vi "Subvi AO trigger.vi"(6 "EnableAsyncTrig":bool, 8 "FrameDelay_tick":u32, 9 "FirstFrameDelay_tick":u32, 10 "Reset":bool, 11 "Trigger":bool) -> (1 "IteratorDirection":bool, 3 "Stop":bool, 4 "Framecount":u16)   [LabVIEW 2017]
uses:
  GV AsyncTrigger.vi
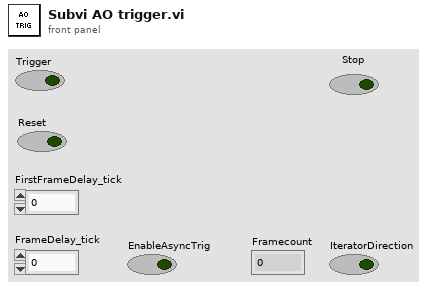
[diagram p1: front panel]
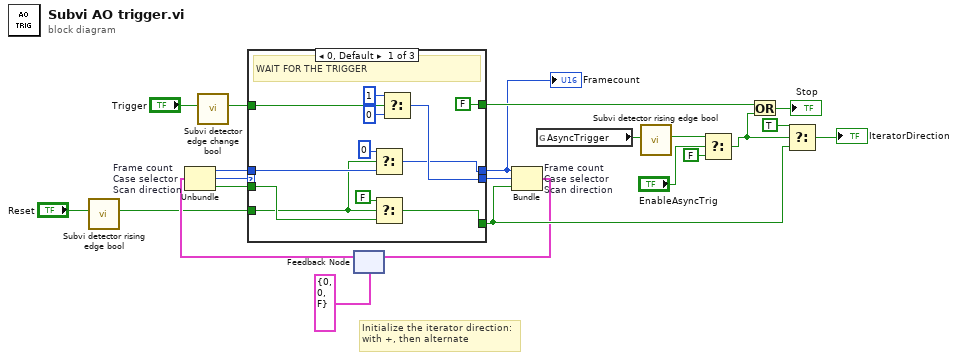
[diagram p0: block diagram]
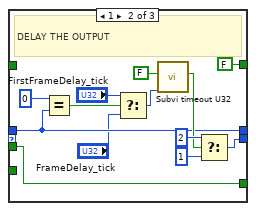
[diagram p2: hidden frame]
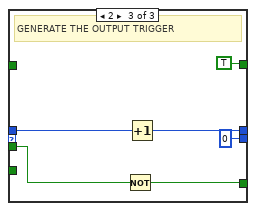
[diagram p3: hidden frame]
diagram:
  # "Initialize the iterator direction:\nwith +, then alternate"
  n1 = call "Subvi detector rising edge bool.vi"("Input"="Reset") -> ("Output"=w6:bool)  [unwired: 10 in]
  n2 = call "Subvi detector edge change bool.vi"("Input"="Trigger") -> ("Output"=w14:bool)  [unwired: 8 in]
  n3 = feedback #1(cluster{i16, "f":u8, bool} {0, "f"=0, FALSE}) -> (w12:cluster{u16, "f":u8, "t":bool})
  n4 = Unbundle "Frame count\nCase selector\nScan direction"(w12) -> (w11:u16, "f"=w9:u8, "t"=w10:bool)
  n5 = case shown="0, Default" w9 {
    tunnel: [w34 w45 u8 0 ("f")] -> w20
    tunnel: [FALSE FALSE TRUE] -> w16
    tunnel: [w26 w43 w51] -> w17
    tunnel: w14 -> [w30 _ _]
    tunnel: [w24 w37 w48] -> w7
    tunnel: w10 -> [w28 w43 w50]
    tunnel: w11 -> [w25 w37 w49]
    tunnel: w6 -> [w23 _ _]
    frame 0, Default {
      # "WAIT FOR THE TRIGGER"
      n6 = Select(t=u16 0, s=w23, f=w25) -> (s? t:f=w24:u16)
      n7 = Select(t=FALSE, s=w23, f=w28) -> (s? t:f=w26:bool)
      n8 = Select(t=u8 1, s=w30, f=u8 0) -> (s? t:f=w34:u8)
    }
    frame 1 {
      # "DELAY THE OUTPUT"
      n9 = Equal?(x=u16 0, y=w37) -> (x = y?=w40:bool)
      n10 = Select(t="FirstFrameDelay_tick", s=w40, f="FrameDelay_tick") -> (s? t:f=w39:u32)
      n11 = call "Subvi timeout U32.vi"("Timeout_tick"=w39, "Input"=FALSE) -> ("Timeout"=w41:bool)  [unwired: 9 in]
      n12 = Select(t=u8 2, s=w41, f=u8 1) -> (s? t:f=w45:u8)
    }
    frame 2 {
      # "GENERATE THE OUTPUT TRIGGER"
      n13 = Not(x=w50) -> (.not. x?=w51:bool)
      n14 = Increment(x=w49) -> (x+1=w48:u16)
    }
  }
  "Framecount" <- w7
  n15 = Bundle "Frame count\nCase selector\nScan direction"(w7, "f"=w20, "t"=w17) -> (w13:cluster{u16, "f":u8, "t":bool})  [unwired: 1 in]
  n16 = feedback-in #1(w13) -> ()
  n17 = global read "GV AsyncTrigger.vi" "AsyncTrigger"() -> (w22:bool)
  n18 = call "Subvi detector rising edge bool.vi"("Input"=w22) -> ("Output"=w4:bool)  [unwired: 10 in]
  n19 = Select(t=w4, s="EnableAsyncTrig", f=FALSE) -> (s? t:f=w3:bool)
  n20 = Or(x=w16, y=w3) -> (x .or. y?=→"Stop":bool)
  n21 = Select(t=TRUE, s=w3, f=w17) -> (s? t:f=→"IteratorDirection":bool)
